vi "INDEX - Tree Control.vi"() -> ()   [LabVIEW 2014, in "DSLV_Tree.lvlib"]
uses:
  DSLV_Tree.lvlib
panel:
  in  "Tree":string(tree)
  # "SEE BLOCK DIAGRAM FOR INDEX"
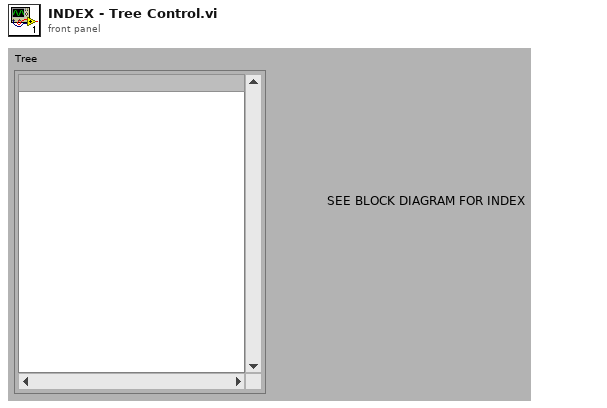
[diagram p1: front panel]
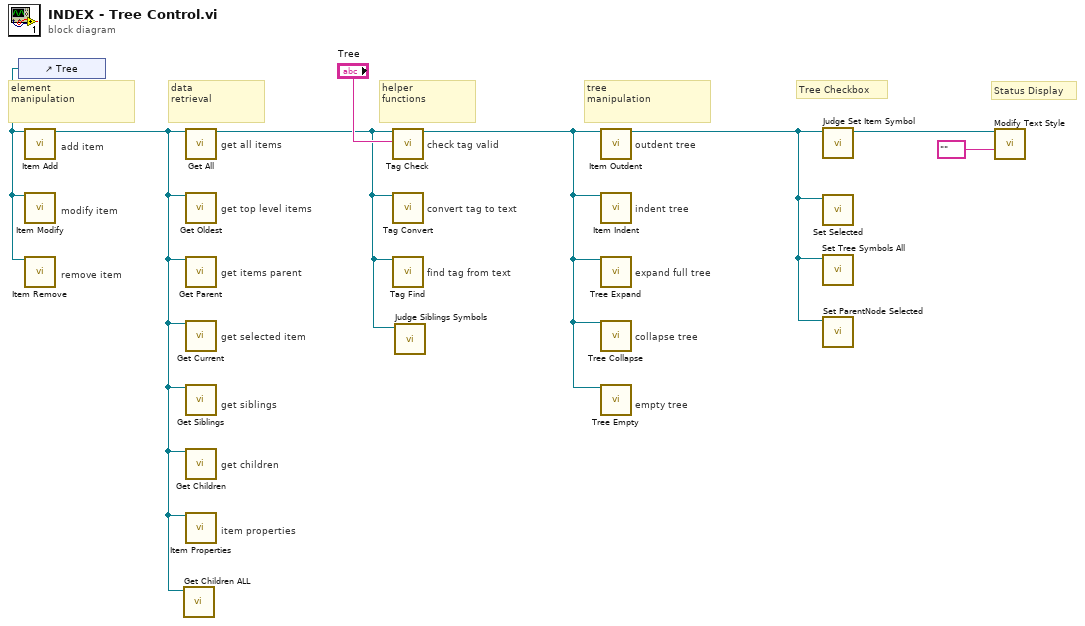
[diagram p0: block diagram]
diagram:
  # "Status Display"
  # "Tree Checkbox"
  # "empty tree"
  # "collapse tree"
  # "expand full tree"
  # "indent tree"
  # "outdent tree"
  # "find tag from text"
  # "convert tag to text"
  # "check tag valid"
  # "get children"
  # "get siblings"
  # "get selected item"
  # "get items parent"
  # "get top level items"
  # "get all items"
  # "item properties"
  # "remove item"
  # "modify item"
  # "add item"
  # "tree\nmanipulation"
  # "helper\nfunctions"
  # "data\nretrieval"
  # "element\nmanipulation"
  n1 = control-ref of="Tree"() -> (w7:refnum<vi>)
  n2 = call "Item Add.vi"("Tree Reference In"=w7) -> ("Tree Reference Out"=w5:refnum<vi>)  [unwired: 16 in, 2 out]
  n3 = call "Item Modify.vi"("Tree Reference In"=w7) -> ()  [unwired: 17 in, 2 out]
  n4 = call "Item Remove.vi"("Tree Reference In"=w7) -> ()  [unwired: 17 in, 2 out]
  n5 = call "Get Children ALL.vi"("Tree Reference"=w5) -> ()  [unwired: 8 in, 3 out]
  n6 = call "Get All.vi"("Tree Reference In"=w5) -> ("Tree Reference Out"=w4:refnum<vi>)  [unwired: 15 in, 3 out]
  n7 = call "Get Oldest.vi"("Tree Reference In"=w5) -> ()  [unwired: 16 in, 3 out]
  n8 = call "Get Parent.vi"("Tree Reference In"=w5) -> ()  [unwired: 15 in, 4 out]
  n9 = call "Get Current.vi"("Tree Reference In"=w5) -> ()  [unwired: 15 in, 4 out]
  n10 = call "Get Siblings.vi"("Tree Reference In"=w5) -> ()  [unwired: 16 in, 3 out]
  n11 = call "Get Children.vi"("Tree Reference In"=w5) -> ()  [unwired: 16 in, 3 out]
  n12 = call "Item Properties.vi"("Tree Reference In"=w5) -> ()  [unwired: 13 in, 6 out]
  n13 = call "Tag Check.vi"("Tree Reference In"=w4, "Input Tag"="Tree") -> ("Tree Reference Out"=w8:refnum<vi>)  [unwired: 14 in, 3 out]
  n14 = call "Tag Convert.vi"("Tree Reference In"=w4) -> ()  [unwired: 15 in, 4 out]
  n15 = call "Tag Find.vi"("Tree Reference In"=w4) -> ()  [unwired: 15 in, 4 out]
  n16 = call "Judge Siblings Symbols.vi"("TreeControl in"=w4) -> ()  [unwired: 8 in, 3 out]
  n17 = call "Item Outdent.vi"("Tree Reference In"=w8) -> ("Tree Reference Out"=w3:refnum<vi>)  [unwired: 17 in, 1 out]
  n18 = call "Item Indent.vi"("Tree Reference In"=w8) -> ()  [unwired: 17 in, 2 out]
  n19 = call "Tree Expand.vi"("Tree Reference In"=w8) -> ()  [unwired: 17 in, 2 out]
  n20 = call "Tree Collapse.vi"("Tree Reference In"=w8) -> ()  [unwired: 17 in, 2 out]
  n21 = call "Tree Empty.vi"("Tree Reference In"=w8) -> ()  [unwired: 16 in, 3 out]
  n22 = call "Judge Set Item Symbol.vi"("TreeControl in"=w3) -> ("TreeControl out"=w2:refnum<vi>)  [unwired: 6 in, 4 out]
  n23 = call "Set Selected.vi"("Tree Reference"=w3) -> ()  [unwired: 8 in, 3 out]
  n24 = call "Set Tree Symbols All.vi"("Tree Refnum"=w3) -> ()  [unwired: 8 in, 3 out]
  n25 = call "Set ParentNode Selected.vi"("TreeControl in"=w3) -> ()  [unwired: 8 in, 3 out]
  n26 = call "Modify Text Style.vi"("Status"="", "Tree Reference"=w2) -> ()  [unwired: 8 in, 2 out]
